vi "MainStartUpSequence.vi"(2 "IntGraph Refnum":refnum<vi>, 5 "error in (no error)":errorcluster) -> (14 "Area":dbl[][](graph), 17 "Point":dbl[][](graph), 19 "error out":errorcluster)   [LabVIEW 2013]
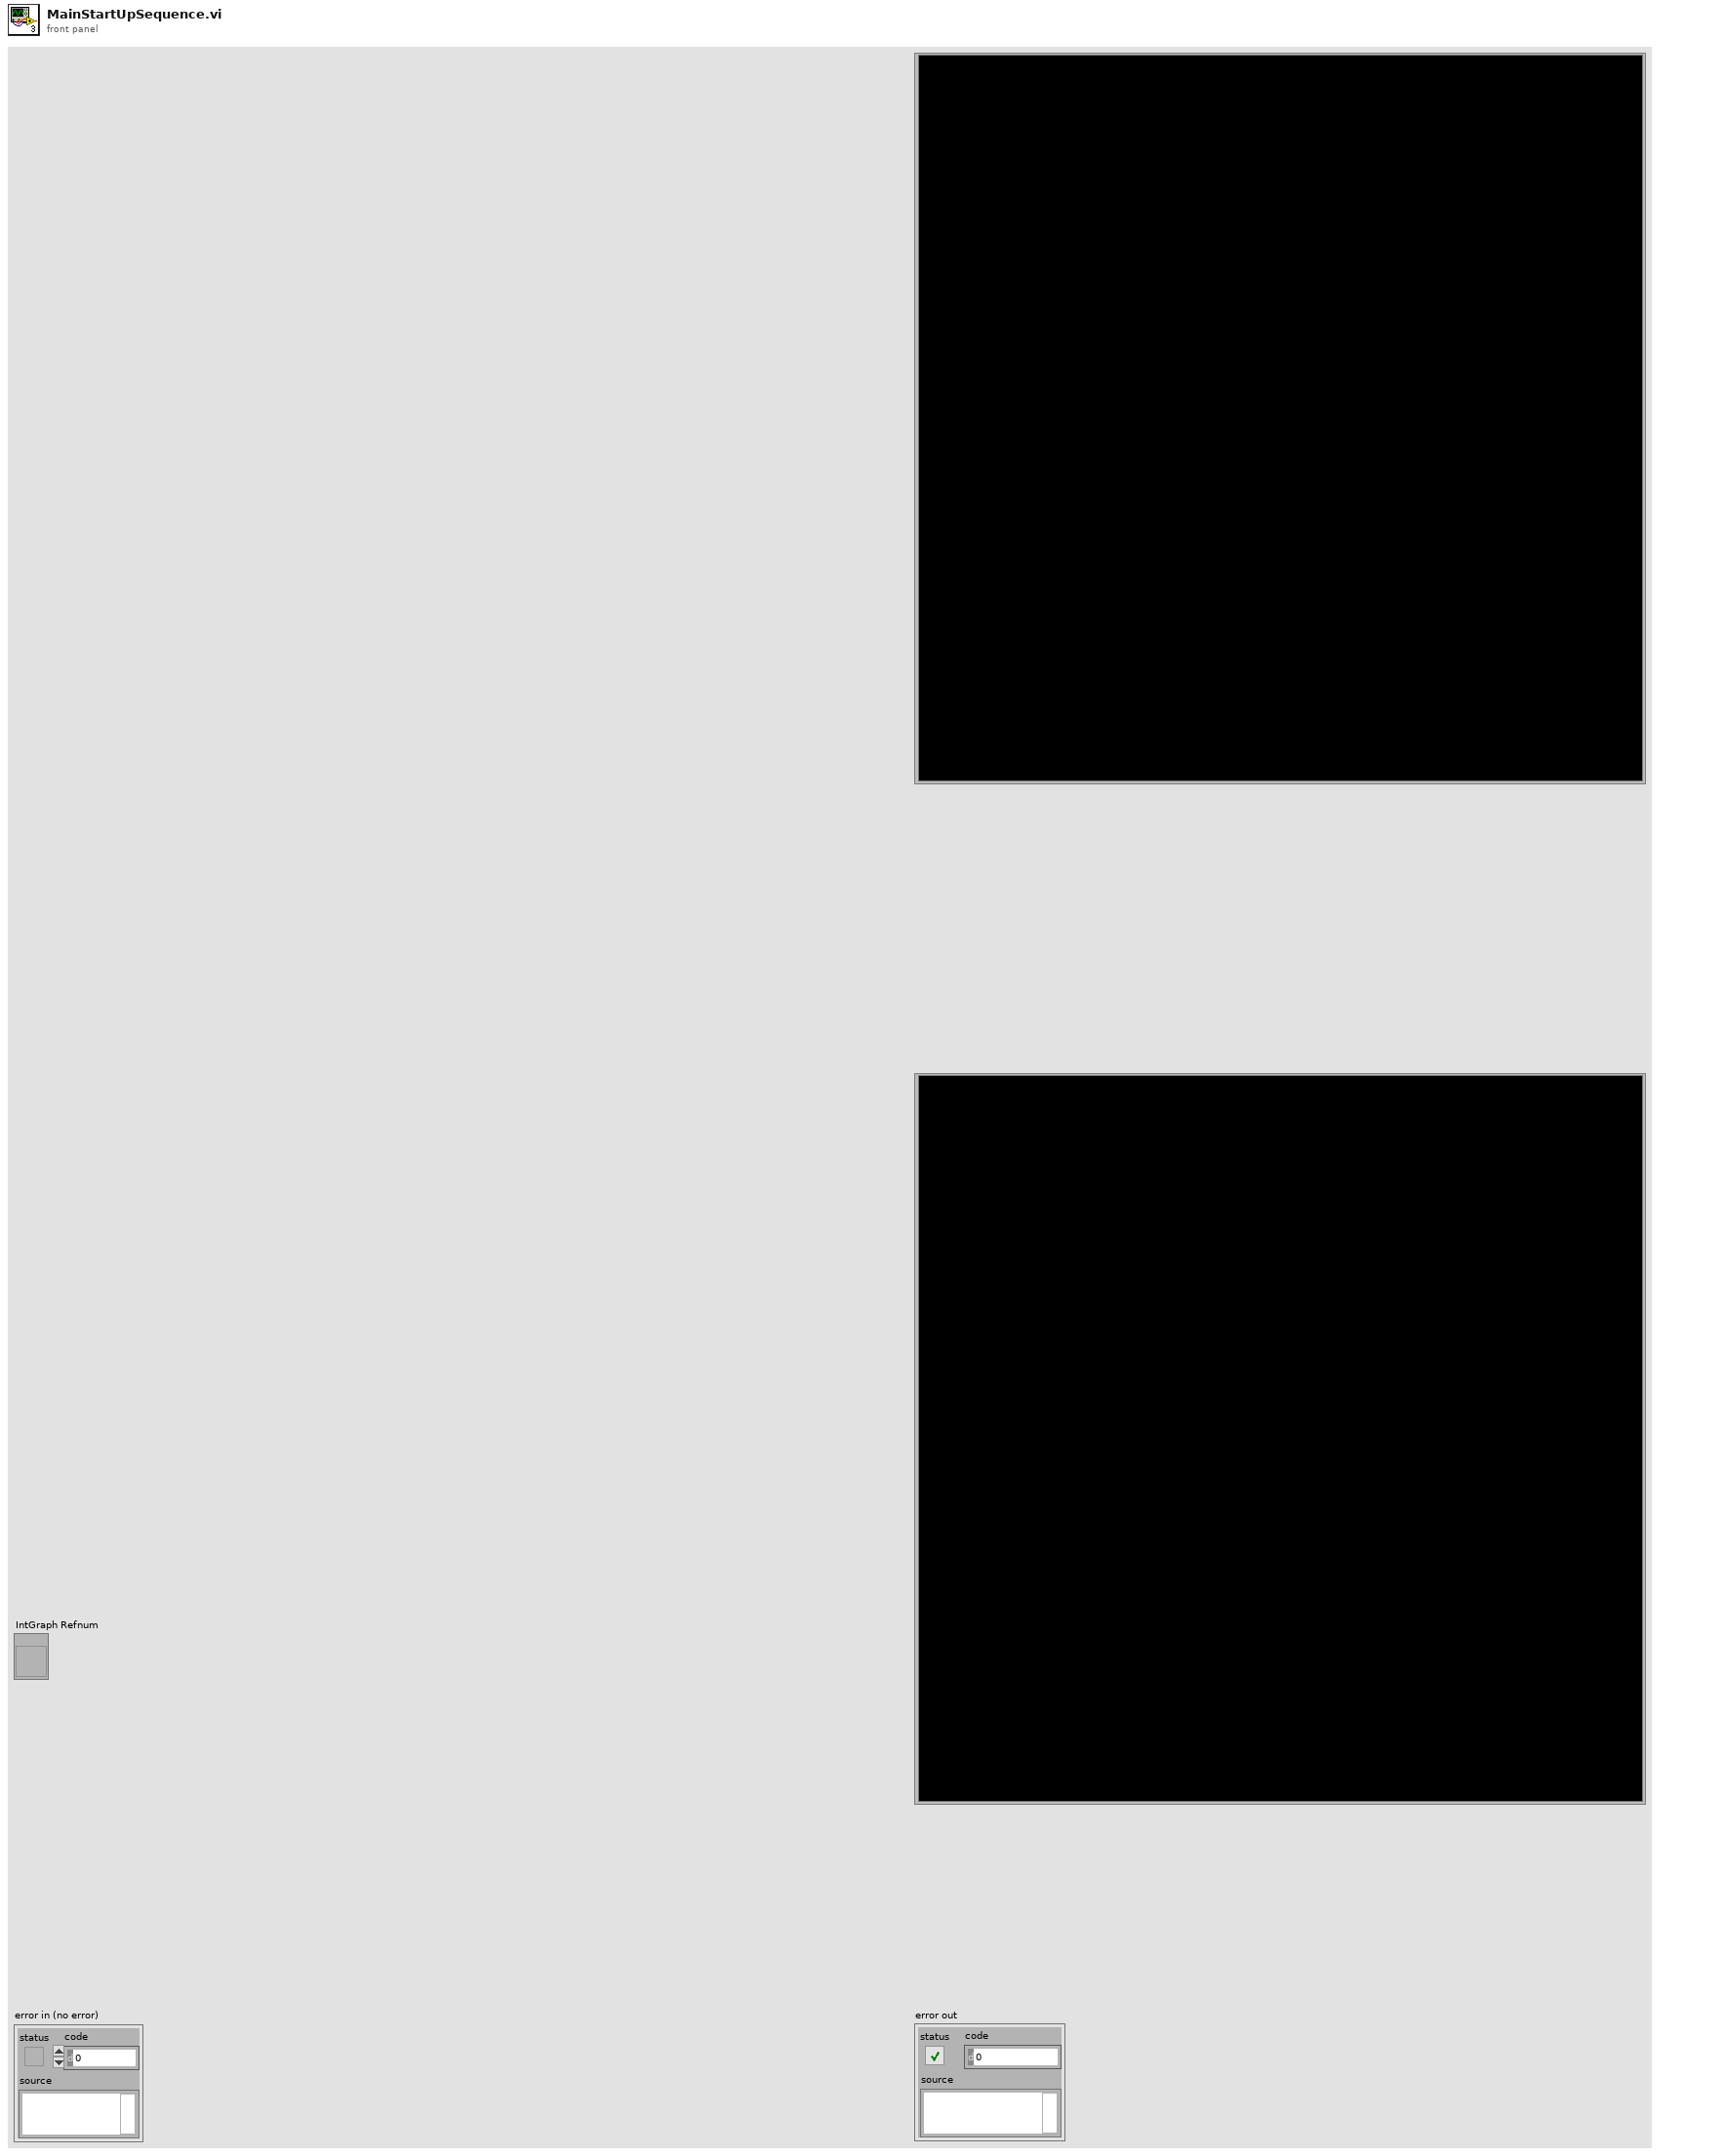
[diagram p1: front panel]
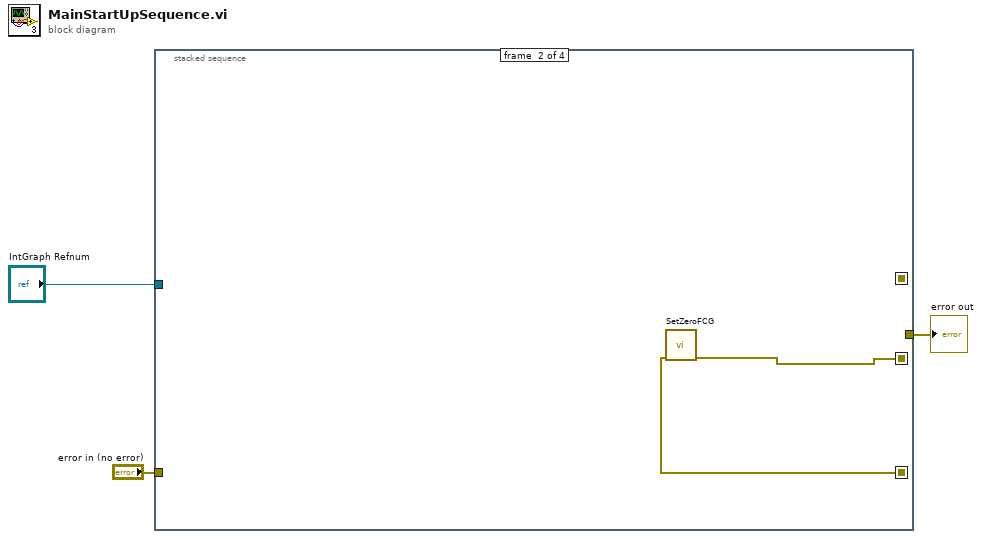
[diagram p0: block diagram]
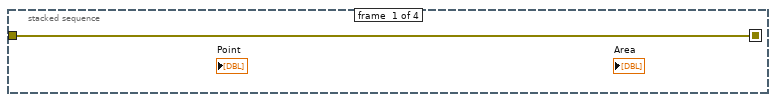
[diagram p2: hidden frame]
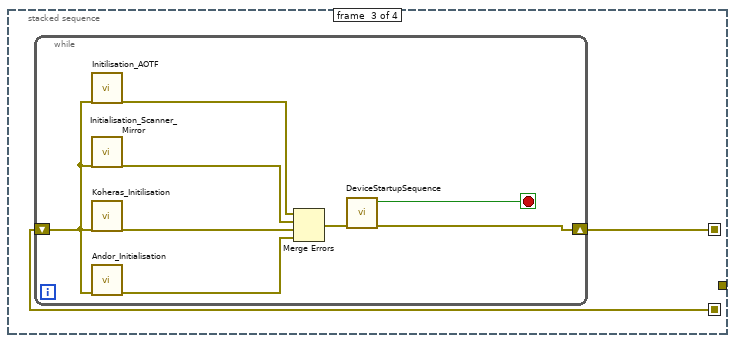
[diagram p3: hidden frame]
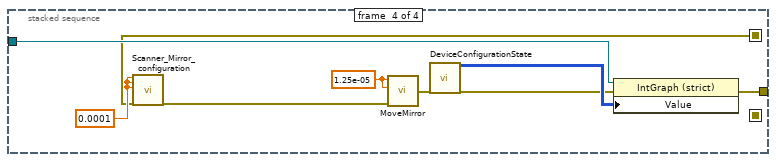
[diagram p4: hidden frame]
diagram:
  n1 = stacked-sequence {
    seq-local: [w4 _ _ _] -> [_ w6 _ _]
    seq-local: [_ w5 _ _] -> [_ _ w8 _]
    seq-local: [_ _ w7 _] -> [_ _ _ w18]
    tunnel: "error in (no error)" -> [w4 _ _ _]
    tunnel: "IntGraph Refnum" -> [_ _ _ w19]
    tunnel: [_ _ _ w17] -> w1
    frame #0 {
    }
    frame #1 {
      n2 = call "SetZeroFCG.vi"("error in (no error)"=w6) -> ("error out"=w5:errorcluster)  [unwired: 10 in]
    }
    frame #2 {
      n3 = while {
        shift-right: [w9] -> w7
        shift-left: w8 -> [w10]
        stop <- w11 stop-if-true
        n4 = call "Initilisation_AOTF.vi"("error in"=w10) -> ("error out"=w15:errorcluster)  [unwired: 18 in]
        n5 = call "Initialisation_Scanner_Mirror.vi"("error in"=w10) -> ("error out"=w14:errorcluster)  [unwired: 18 in]
        n6 = call "Koheras_Initilisation.vi"("error in"=w10) -> ("error out"=w13:errorcluster)  [unwired: 18 in]
        n7 = call "Andor_Initialisation.vi"("error in (no error)"=w10) -> ("error out"=w12:errorcluster)  [unwired: 10 in]
        n8 = Merge Errors(w15, w14, w13, w12) -> (w16:errorcluster)
        n9 = call "DeviceStartupSequence.vi"("error in"=w16) -> ("error out"=w9:errorcluster, "DeviceStartUpDone"=w11:bool)  [unwired: 9 in]
      }
    }
    frame #3 {
      w20 = 1.25e-05 ("POS Y rad")
      w21 = 0.0001 ("POS X")
      n10 = call "Scanner_Mirror_configuration.vi"("POS X"=w21, "POS Y"=w21, "POS Z"=w21, "error in"=w18) -> ("error out"=w23:errorcluster)  [unwired: 15 in]
      n11 = call "MoveMirror.vi"("error in 2"=w23, "POS X rad"=w20, "POS Y rad"=w20) -> ("error out 2"=w22:errorcluster)  [unwired: 1 in]
      n12 = call "DeviceConfigurationState.vi"("error out"=w22) -> ("image"=w25:i32[][], "error out 2"=w24:errorcluster)  [unwired: 17 in]
      n13 = property on="Property Node" class="IntGraph (strict)"(reference=w19, error in=w24, "Value"=w25) -> (error out=w17:errorcluster)  [unwired: 1 out]
    }
  }
  "error out" <- w1
